vi "Tone RMS from Mag Spec.vi"(8 "error in (no error)":errorcluster, 9 "Gain":dbl, 10 "Frequency (Hz)":dbl[](array[numeric]), 11 "Magnitude (dB)":dbl[](array[numeric])) -> (0 "error out":errorcluster, 1 "Fpeak":dbl, 2 "RMS (dB)":dbl, 3 "RMS (V)":dbl)   [LabVIEW 2020]
uses:
  3118ad97-552b-4e98-9a50-97e7f1a9a5d7.vi
  4471f674-7cfa-43e3-aef7-e2e44c13a995.vi
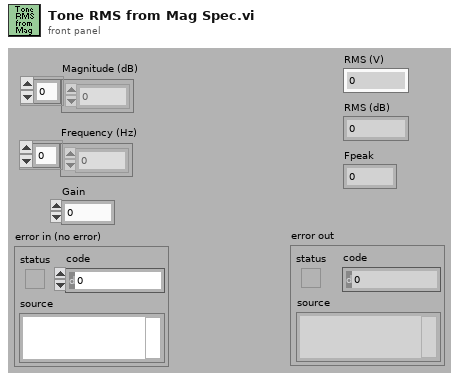
[diagram p1: front panel]
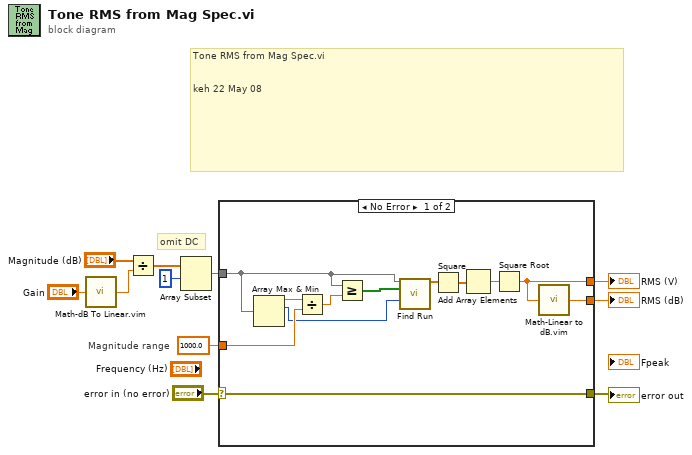
[diagram p0: block diagram]
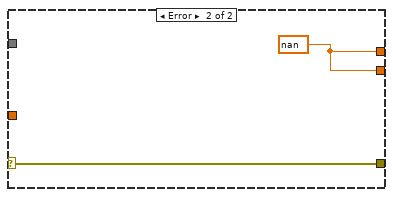
[diagram p2: hidden frame]
diagram:
  # "omit DC"
  # "Magnitude range"
  # "Tone RMS from Mag Spec.vi\n\n\nkeh 22 May 08"
  n1 = call "Math-dB To Linear.vim"("dB"="Gain") -> ("linear"=w2:dbl)
  n2 = Divide(x="Magnitude (dB)", y=w2) -> (x/y=w5:dbl[])
  n3 = Array Subset(array=w5, index=1) -> (w6:dbl[])  [unwired: 1 in]
  n4 = case shown="No Error" "error in (no error)" {
    selector: "error in (no error)" -> [w18 w25]
    tunnel: w6 -> [w16 _]
    tunnel: 1000.0 -> [w22 _]
    tunnel: [w12 w24] -> w9
    tunnel: [w18 w25] -> w8
    tunnel: [w17 w24] -> w1
    frame No Error {
      n5 = Array Max & Min(array=w16) -> (max value=w23:dbl, max index (indices)=w19:i32)  [unwired: 2 out]
      n6 = Divide(x=w23, y=w22) -> (x/y=w21:dbl)
      n7 = Greater Or Equal?(x=w16, y=w21) -> (x >= y?=w20:bool[])
      n8 = call "Find Run.vi"("Array"=w16, "Condition"=w20, "Midrun index"=w19) -> ("Run"=w15:dbl[])  [unwired: 9 in, 3 out]
      n9 = Square(x=w15) -> (x^2=w14:dbl[])
      n10 = Add Array Elements(numeric array=w14) -> (sum=w13:dbl)
      n11 = Square Root(x=w13) -> (sqrt(x)=w12:dbl)
      n12 = call "Math-Linear to dB.vim"("linear"=w12) -> ("dB"=w17:dbl)
    }
    frame Error {
      w24 = nan
    }
  }
  "error out" <- w8
  "RMS (V)" <- w9
  "RMS (dB)" <- w1
